vi "set_multiramp_soak_segment_event_configuration.vi"(6 "Soak enabled":bool, 8 "error in (no error)":errorcluster, 9 "Ramp enabled":bool, 10 "Segment number":u8 max=15, 11 "VISA Refnum in":refnum<visa-resource-name>) -> (0 "error out":errorcluster, 3 "VISA Refnum out":refnum<visa-resource-name>)   [LabVIEW 2018]
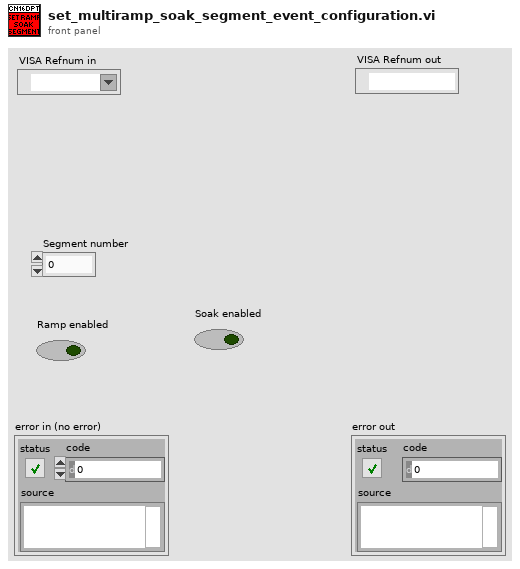
[diagram p1: front panel]
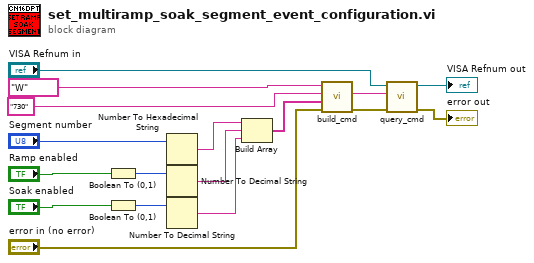
[diagram p0: block diagram]
diagram:
  n1 = Boolean To (0,1)(Boolean="Ramp enabled") -> (0, 1=w7:i16)
  n2 = Boolean To (0,1)(Boolean="Soak enabled") -> (0, 1=w3:i16)
  n3 = Number To Hexadecimal String(2:"Segment number") -> (0:w4:string)  [unwired: 1 in]
  n4 = Number To Decimal String(number=w7) -> (decimal integer string=w6:string)  [unwired: 1 in]
  n5 = Number To Decimal String(number=w3) -> (decimal integer string=w1:string)  [unwired: 1 in]
  n6 = Build Array(w4, w6, w1) -> (w9:string[])
  n7 = call "build_cmd.vi"("error in (no error)"="error in (no error)", "Parameter list"=w9, "Command ID"="730", "Command class"="W") -> ("error out"=w12:errorcluster, "Command"=w11:string)  [unwired: 6 in]
  n8 = call "query_cmd.vi"("error in (no error)"=w12, "Command"=w11, "VISA resource name"="VISA Refnum in") -> ("error out"=→"error out":errorcluster, "VISA resource name out"=→"VISA Refnum out":refnum<visa-resource-name>)  [unwired: 6 in, 1 out]
